vi "gyro_get_flags.vi"(11 "all rows":string[][](array[string])) -> (3 "flag-timestamp array":cluster{"String":string, timestamp}[](array[cluster]))   [LabVIEW 2020]
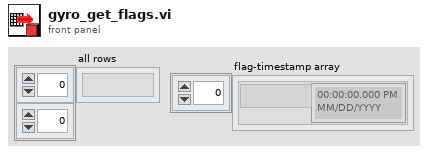
[diagram p1: front panel]
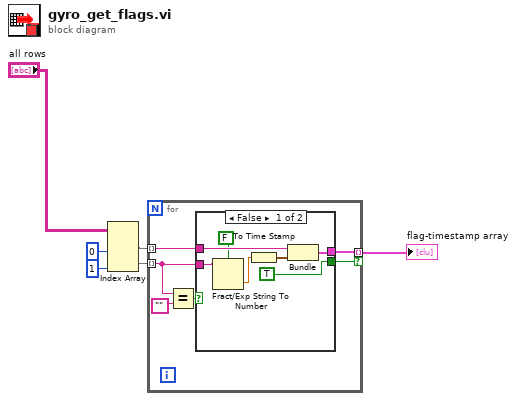
[diagram p0: block diagram]
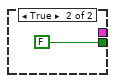
[diagram p2: hidden frame]
diagram:
  n1 = Index Array(array="all rows", index (col) #1=0 ("disabled index (col)"), index (col) #2=1 ("index (col)")) -> (element #1=w5:string[], element #2=w6:string[])  [unwired: 2 in]
  n2 = for {
    tunnel: w5 -> [w10] mode=indexing
    tunnel: w6 -> [w9] mode=indexing
    tunnel: [w8] -> w1 mode=indexing if=w7
    n3 = Equal?(x=w9, y="") -> (x = y?=w11:bool)
    n4 = case shown="False" w11 {
      tunnel: w10 -> [w16 _]
      tunnel: w9 -> [w19 _]
      tunnel: [w18 _] -> w8
      tunnel: [TRUE FALSE] -> w7
      frame False {
        n5 = Fract/Exp String To Number(use system decimal point (T)=FALSE, string=w19) -> (number=w15:dbl)  [unwired: 2 in, 1 out]
        n6 = To Time Stamp(1:w15) -> (0:w14:timestamp)
        n7 = Bundle("String"=w16, w14) -> (w18:cluster{"String":string, timestamp})  [unwired: 1 in]
      }
      frame True {
      }
    }
  }
  "flag-timestamp array" <- w1
